vi "GetControlsAndIndicatorNames.vi"(8 "error in (no error)":errorcluster, 11 "VI Refnum":refnum<vi>) -> (0 "error out":errorcluster, 1 "Indicators":string[](array[string]), 2 "Controls":string[](array[string]), 3 "VI Refnum out":refnum<vi>)   [LabVIEW 2015]
doc: "This VI retrieves the names of all indicators and all controls from the VI referenced."
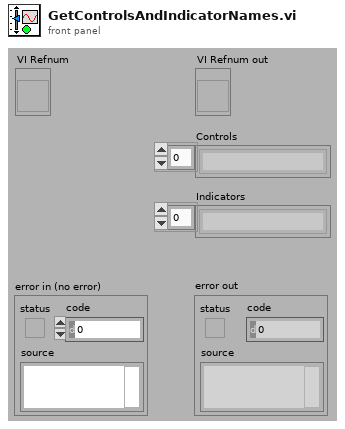
[diagram p1: front panel]
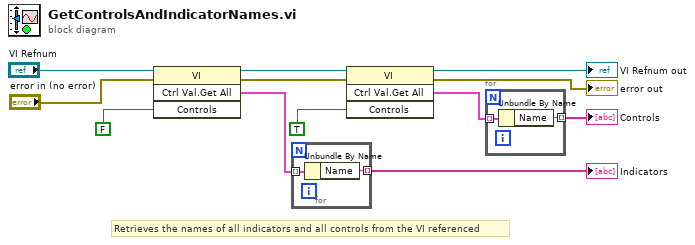
[diagram p0: block diagram]
diagram:
  # "Retrieves the names of all indicators and all controls from the VI referenced"
  n1 = invoke class="VI" method="Ctrl Val.Get All"(reference="VI Refnum", error in="error in (no error)", "Controls"=FALSE) -> (reference out=w7:refnum<vi>, error out=w8:errorcluster, "Get All Control Values Variant"=w10:cluster{"Name":string, "Variant Data":variant}[])  [unwired: 1 in, 1 out]
  n2 = for {
    tunnel: w10 -> [w14] mode=indexing
    tunnel: [w13] -> w1 mode=indexing
    n3 = Unbundle By Name(w14) -> ("Name"=w13:string)
  }
  "Indicators" <- w1
  n4 = invoke class="VI" method="Ctrl Val.Get All"(reference=w7, error in=w8, "Controls"=TRUE) -> (reference out=→"VI Refnum out":refnum<vi>, error out=→"error out":errorcluster, "Get All Control Values Variant"=w9:cluster{"Name":string, "Variant Data":variant}[])  [unwired: 1 in, 1 out]
  n5 = for {
    tunnel: w9 -> [w16] mode=indexing
    tunnel: [w15] -> w2 mode=indexing
    n6 = Unbundle By Name(w16) -> ("Name"=w15:string)
  }
  "Controls" <- w2
